vi "Write LSEConfig.vi"(8 "error in (no error)":errorcluster, 10 "LSEConfig":T1={"NoiseVariance"=0.0, "IEEESystem"=39, "PMULocations"=[16], "Vindex"=0, "Iindex"=3, "DynamicRef"=""}, 11 "LSEPlugin in":refnum<class "LSEPlugin.lvclass">) -> (0 "error out":errorcluster, 3 "LSEPlugin out":refnum<class "LSEPlugin.lvclass">)   [LabVIEW 2017, in "AppPlugins.lvlib" / "LSEPlugin.lvclass"]
uses:
  LSEPlugin.lvclass
  PublicAPI/Typedefs/LSEConfig.ctl
  LSEPlugin.lvclass/LSEPlugin.ctl
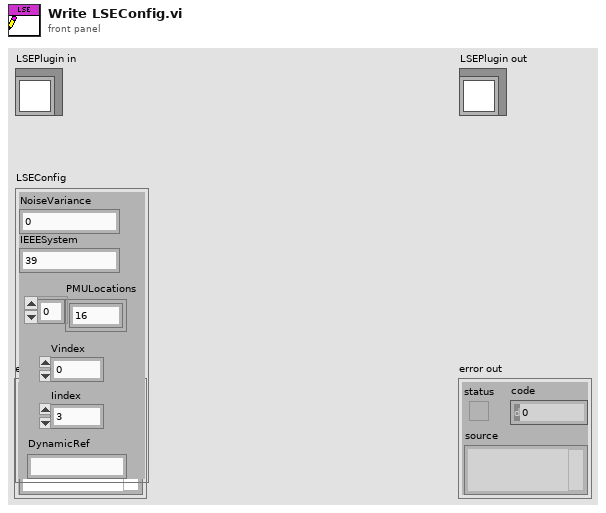
[diagram p1: front panel]
types:
  T1 = typedef "AppPlugins.lvlib/LSEPlugin.lvclass/LSEConfig.ctl" = cluster{"NoiseVariance":dbl, "IEEESystem":u32, "PMULocations":u32[], "Vindex":i32, "Iindex":i32, "DynamicRef":string}
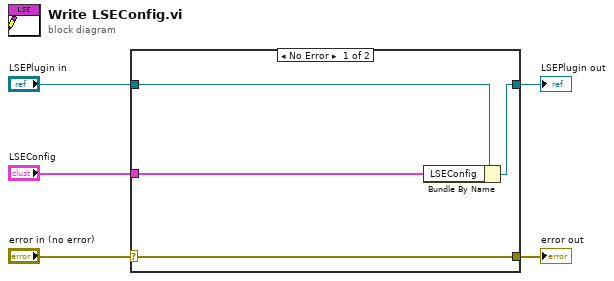
[diagram p0: block diagram]
diagram:
  n1 = case shown="No Error" "error in (no error)" {
    selector: "error in (no error)" -> [w9 w10]
    tunnel: [w9 w10] -> w4
    tunnel: [w7 w11] -> w2
    tunnel: "LSEPlugin in" -> [w8 w11]
    tunnel: "LSEConfig" -> [w6 _]
    frame No Error {
      n2 = Bundle By Name(cluster=w8, "LSEConfig"=w6) -> (w7:refnum<class "LSEPlugin.lvclass">)
    }
    frame Error {
    }
  }
  "error out" <- w4
  "LSEPlugin out" <- w2
